vi "ROI group-Delete groups from all groups FG.vi"(8 "error in (no error)":errorcluster, 11 "Names of groups to delete":string[](array[string])) -> (0 "error out":errorcluster, 2 "Updated groups setup":T1[](array[typedef]) {"Group region specifier cluster"."Contours"."Type" items=["No Selection", "Point", "Line", "Rectangle", "Oval", "Polygon", "Freehand Region", "Annulus", "Unused2", "Unused3", "Broken Line", "Freehand Line", "Rotated Rectangle"]})   [LabVIEW 2017]
uses:
  ROI Selection Interface/ROI group info cluster.ctl
  Typedefs/Get-Set-Clear Control.ctl
  <userlib>/_OpenG.lib/array/array.llb/Delete Elements from 1D Array (Variant)__ogtk.vi
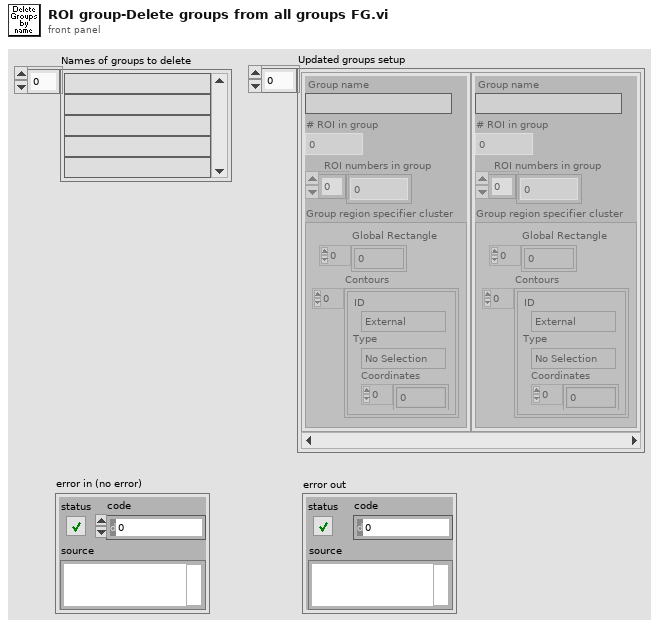
[diagram p1: front panel]
types:
  T1 = typedef "ROI group info cluster.ctl" = cluster{"Group name":string, "# ROI in group":i32, "ROI numbers in group":i32[], "Group region specifier cluster":T2}
  T2 = typedef "ROI Descriptor" = cluster{"Global Rectangle":i32[], "Contours":cluster{"ID":enum32{"External", "Internal"}, "Type":u32, "Coordinates":i32[]}[]}
  T3 = typedef "Get-Set-Clear Control.ctl" = enum16{"Get", "Set", "Clear"}
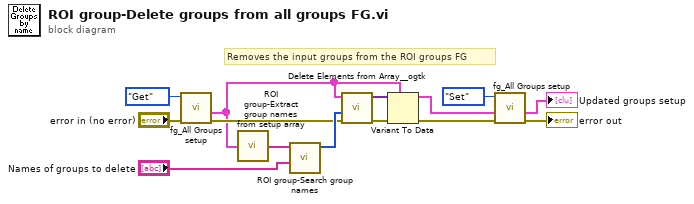
[diagram p0: block diagram]
diagram:
  # "Removes the input groups from the ROI groups FG"
  n1 = call "fg_All Groups setup.vi"("error in (no error)"="error in (no error)", "Function"=Get-Set-Clear_Control."Get") -> ("error out"=w5:errorcluster, "Groups setup out"=w1:T1[])  [unwired: 8 in]
  n2 = call "ROI group-Extract group names from setup array.vi"("Groups setup"=w1) -> ("Group Names Array"=w8:string[])
  n3 = call "ROI group-Search group names.vi"("Group names to search for"="Names of groups to delete", "Group names to search through"=w8) -> ("Indexes (-1 = not found)"=w11:i32[])  [unwired: 9 in]
  n4 = call-poly <userlib>:"Delete Elements from Array__ogtk.vi"("indices"=w11, "array"=w1) -> ("array w/ subset deleted"=w10:variant[])  [unwired: 8 in, 1 out]
  n5 = Variant To Data(error in=w5, type=w1, Variant=w10) -> (data=w9:T1[], error out=w3:errorcluster)
  n6 = call "fg_All Groups setup.vi"("error in (no error)"=w3, "Groups setup in"=w9, "Function"=Get-Set-Clear_Control."Set") -> ("error out"=→"error out":errorcluster, "Groups setup out"=→"Updated groups setup":T1[])  [unwired: 7 in]
